vi "Read INI File.vi"(8 "error in (no error)":errorcluster, 11 "Terminal Menus in":refnum<class "Terminal Menus.lvclass">) -> (0 "error out":errorcluster, 3 "Terminal Menus out":refnum<class "Terminal Menus.lvclass">)   [LabVIEW 2016, in "CLD Exam - ATM.lvlib" / "Terminal Menus.lvclass"]
uses:
  Terminal Menus.lvclass
  Terminal Menus.lvclass/Terminal Menus.ctl
  <vilib>/Utility/config.llb/Read Key (String).vi
  <vilib>/Utility/config.llb/NI_LVConfig.lvlib
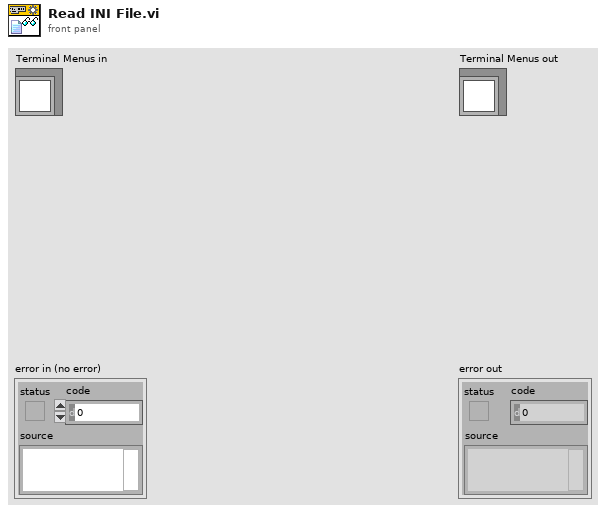
[diagram p1: front panel]
types:
  T1 = typedef "NI_LVConfig.lvlib/Config Data RefNum.ctl" = refnum<k1>
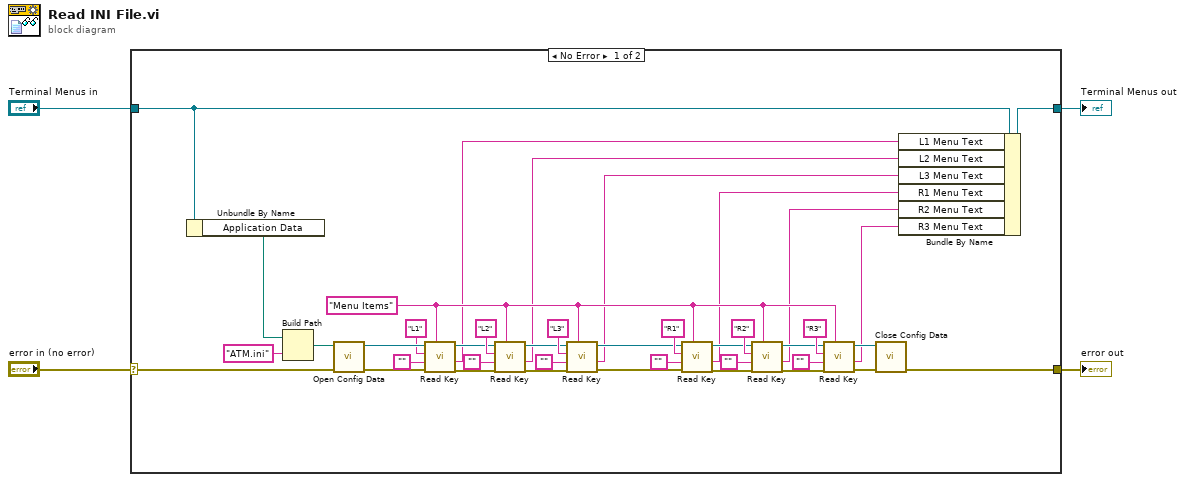
[diagram p0: block diagram]
diagram:
  n1 = case shown="No Error" "error in (no error)" {
    selector: "error in (no error)" -> [w15 w46]
    tunnel: [w14 w46] -> w3
    tunnel: [w11 w45] -> w1
    tunnel: "Terminal Menus in" -> [w12 w45]
    frame No Error {
      w24 = "Menu Items" ("section")
      n2 = Unbundle By Name(w12) -> ("Application Data"=w13:path)
      n3 = Build Path(base path=w13, name or relative path="ATM.ini") -> (appended path=w44:path)
      n4 = call <vilib>:"Open Config Data.vi"("error in (no error)"=w15, "configuration file path"=w44) -> ("error out"=w41:errorcluster, "refnum"=w42:T1)  [unwired: 7 in, 1 out]
      n5 = call-poly <vilib>:"Read Key.vi"("section"=w24, "error in (no error)"=w41, "default value"="", "key"="L1", "refnum"=w42) -> ("error out"=w34:errorcluster, "value"=w10:string, "refnum out"=w22:T1)  [unwired: 3 in, 1 out]
      n6 = call-poly <vilib>:"Read Key.vi"("section"=w24, "error in (no error)"=w34, "default value"="", "key"="L2", "refnum"=w22) -> ("error out"=w33:errorcluster, "value"=w9:string, "refnum out"=w21:T1)  [unwired: 3 in, 1 out]
      n7 = call-poly <vilib>:"Read Key.vi"("section"=w24, "error in (no error)"=w33, "default value"="", "key"="L3", "refnum"=w21) -> ("error out"=w23:errorcluster, "value"=w8:string, "refnum out"=w20:T1)  [unwired: 3 in, 1 out]
      n8 = call-poly <vilib>:"Read Key.vi"("section"=w24, "error in (no error)"=w23, "default value"="", "key"="R1", "refnum"=w20) -> ("error out"=w31:errorcluster, "value"=w7:string, "refnum out"=w19:T1)  [unwired: 3 in, 1 out]
      n9 = call-poly <vilib>:"Read Key.vi"("section"=w24, "error in (no error)"=w31, "default value"="", "key"="R2", "refnum"=w19) -> ("error out"=w32:errorcluster, "value"=w6:string, "refnum out"=w18:T1)  [unwired: 3 in, 1 out]
      n10 = call-poly <vilib>:"Read Key.vi"("section"=w24, "error in (no error)"=w32, "default value"="", "key"="R3", "refnum"=w18) -> ("error out"=w16:errorcluster, "value"=w5:string, "refnum out"=w17:T1)  [unwired: 3 in, 1 out]
      n11 = call <vilib>:"Close Config Data.vi"("error in (no error)"=w16, "refnum"=w17) -> ("error out"=w14:errorcluster)  [unwired: 8 in, 1 out]
      n12 = Bundle By Name(cluster=w12, "L1 Menu Text"=w10, "L2 Menu Text"=w9, "L3 Menu Text"=w8, "R1 Menu Text"=w7, "R2 Menu Text"=w6, "R3 Menu Text"=w5) -> (w11:refnum<class "Terminal Menus.lvclass">)
    }
    frame Error {
    }
  }
  "error out" <- w3
  "Terminal Menus out" <- w1
